vi "ActionVIOnDelete.vi"(6 "All deleted Refs":T1[](array[typedef]) format="%.0x", 8 "error in (no error)":errorcluster, 11 "Item Ref in":T1 format="%.0x") -> (0 "error out":errorcluster, 3 "Item Ref out":T1 format="%.0x")   [LabVIEW 2019, in "UDP-Custom-Device System Explorer.lvlib"]
uses:
  UDP-Custom-Device System Explorer.lvlib
  <vilib>/NI VeriStand/Custom Device API/Custom Device Item Ref.ctl
  Shared/Constants.vi
  <vilib>/NI VeriStand/Custom Device Tools/Custom Device Utility Library/NI VeriStand - Search for Item by GUID.vi
  <vilib>/NI VeriStand/Custom Device Tools/Custom Device Utility Library/Custom Device Utility Library.lvlib
  Shared/UDP-Custom-Device Shared.lvlib
  <vilib>/NI VeriStand/Custom Device API/Custom Device API.lvlib
  Property Accessors/Shared Section Accessors.lvlib
  Property Accessors/Shared Packet Accessors.lvlib
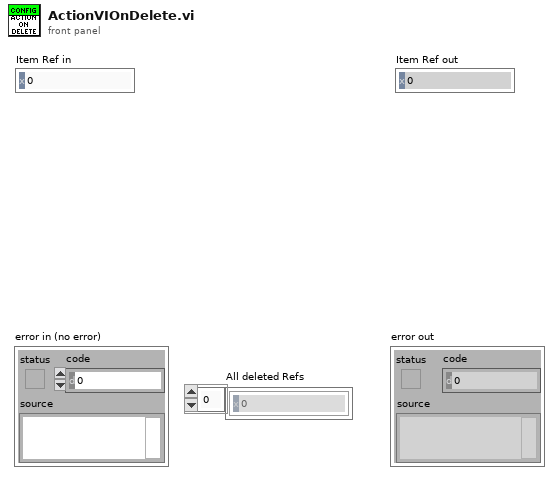
[diagram p1: front panel]
types:
  T1 = typedef "Custom Device API.lvlib/Custom Device Item Ref.ctl" = u64
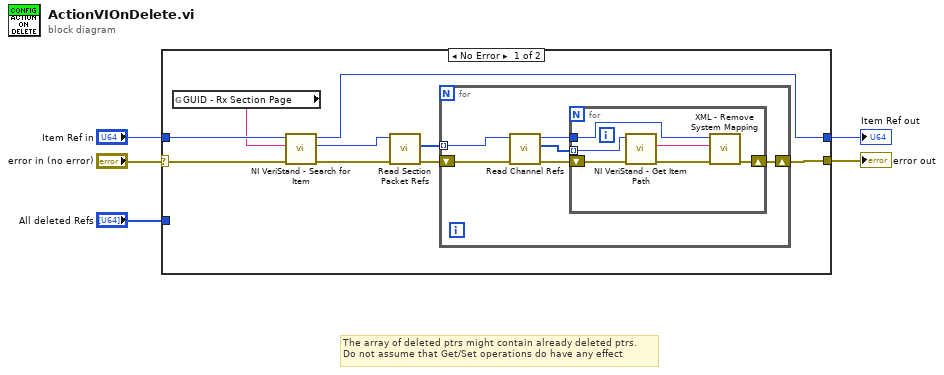
[diagram p0: block diagram]
diagram:
  # "The array of deleted ptrs might contain already deleted ptrs.\nDo not assume that Get/Set operations do have any effect"
  n1 = case shown="No Error" "error in (no error)" {
    selector: "error in (no error)" -> [w13 w28]
    tunnel: [w12 w28] -> w4
    tunnel: "Item Ref in" -> [w14 w27]
    tunnel: [w10 w27] -> w2
    tunnel: "All deleted Refs" -> [_ _]
    frame No Error {
      n2 = global read "Constants.vi" "GUID - Rx Section Page"() -> (w11:string)
      n3 = call-poly <vilib>:"NI VeriStand - Search for Item.vi"("error in"=w13, "Item GUID"=w11, "Section Ref in"=w14) -> ("error out"=w8:errorcluster, "Item Ref"=w9:T1, "Section Ref out"=w10:T1)  [unwired: 5 in, 1 out]
      n4 = call "Read Section Packet Refs.vi"("error in (no error)"=w8, "Node Ptr"=w9) -> ("error out"=w6:errorcluster, "Dependent Node Refs"=w7:T1[])  [unwired: 7 in, 1 out]
      n5 = for {
        tunnel: w7 -> [w19] mode=indexing
        shift-right: [w20] -> w12
        shift-left: w6 -> [w16]
        n6 = call "Read Channel Refs.vi"("error in (no error)"=w16, "Node Ptr"=w19) -> ("error out"=w15:errorcluster, "Dependent Node Refs"=w17:T1[], "Node Ptr out"=w18:T1)  [unwired: 7 in]
        n7 = for {
          shift-right: [w26] -> w20
          shift-left: w15 -> [w23]
          tunnel: w18 -> [w21]
          tunnel: w17 -> [w22] mode=indexing
          n8 = call <vilib>:"NI VeriStand - Get Item Path.vi"("error in (no error)"=w23, "Item Ref in"=w22) -> ("error out"=w25:errorcluster, "Path"=w24:string)  [unwired: 6 in, 2 out]
          n9 = call "XML - Remove System Mapping.vi"("error in (no error)"=w25, "Channel Path Destination"=w24, "Item Ref in"=w21) -> ("error out"=w26:errorcluster)  [unwired: 7 in, 1 out]
        }
      }
    }
    frame Error {
    }
  }
  "error out" <- w4
  "Item Ref out" <- w2
